vi "Write Both Fan States.vi"(8 "error in (no error)":cluster{"状态":bool, "代码":i32, "源":string} caption="错误输入（无错误）", 9 "风扇B状态":bool, 10 "风扇A状态":bool, 11 "仿真双风扇输入":refnum<class "Simulated Dual Fan.lvclass">) -> (0 "error out":cluster{"状态":bool, "代码":i32, "源":string} caption="错误输出")   [LabVIEW 2015, in "Simulated Dual Fan.lvclass"]
uses:
  Simulated Dual Fan.lvclass
  Cooler Plug-Ins/Simulated Evaporative Cooler.lvclass/Simulation Data_Global.vi
  Cooler Plug-Ins/Simulated Evaporative Cooler.lvclass/Simulated Evaporative Cooler.lvclass
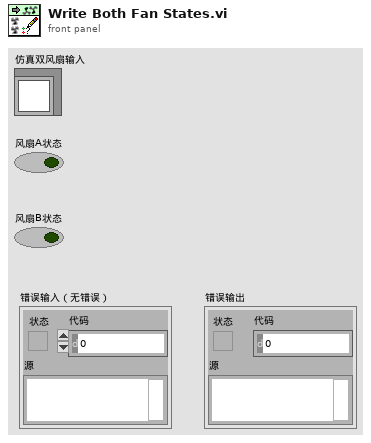
[diagram p1: front panel]
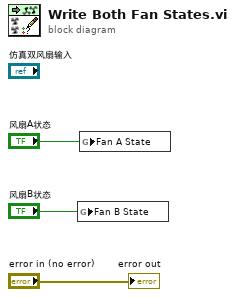
[diagram p0: block diagram]
diagram:
  n1 = global write "Simulation Data_Global.vi" "Fan B State"("风扇B状态") -> ()
  n2 = global write "Simulation Data_Global.vi" "Fan A State"("风扇A状态") -> ()
  "error out" <- "error in (no error)"
